vi "Instrument_Setup.vi"() -> ()   [LabVIEW 2016]
uses:
  sub_vi-s/Equipment/Oxford Software/Oxsoft/PSSUBS.LLB/PSIO.ctl
  sub_vi-s/Equipment/Oxford Software/Oxsoft/BUSGEN.LLB/OxfordAddress.ctl
  sub_vi-s/Equipment/Oxford Software/Oxsoft/ITCSUBS.LLB/ITCIO.ctl
  sub_vi-s/Equipment/Oxford Software/Oxsoft/ITCSUBS.LLB/ITCVersion.ctl
  sub_vi-s/Equipment/Oxford Software/Oxsoft/PSAPPS.LLB/PSSetupArray.ctl
  sub_vi-s/Equipment/Oxford Software/Oxsoft/PSAPPS.LLB/PSSetup.ctl
  sub_vi-s/Equipment/Oxford Software/Oxsoft/ITCAPPS.LLB/ITCSetup.ctl
  sub_vi-s/Equipment/Oxford Software/Oxsoft/LCSUBS.LLB/LambdaSetup.ctl
  sub_vi-s/Equipment/Oxford Software/Oxsoft/Ilmapps.llb/ILMSetup.ctl
panel:
  in  "Registerkarte":T1(tab)=enum."Keithley 6221"
  in  "Insert":string(combo)="VTI"
  in  "Instrument":string(combo)="Sweet 16"
  in  "Temperature control":bool
  in  "Set-Lockin-Sens":u16(ring) items=["Command File", "Auto", "Status Monitor"]
  in  "Logfile folder":path=path "D:/Cryostat Software/Logfiles"
  in  "16 T":bool
  in  "AH 2500":bool
  in  "Set magnet persistent":bool
  in  "Keithley 6221":bool
  in  "readout (s)":dbl=1.0 min=0.0 format="%#_6f"
  in  "LS372 mitloggen":bool
  in  "Stepmodus":enum16{"linear", "1/x", "Logx"}(ring)
  in  "LS370 mitloggen":bool
  in  "Initializiation-File-Folder":path=path "D:/Messdaten/Init-Files"
  in  "Command-File":path=path "D:/Cryostat Software/CryoTUM-V1.0/Command-File.txt"
  in  "Datafile-Folder":path=path "D:/Messdaten"
  in  "Keithley":bool
  in  "Lock In #3":bool
  in  "Lock In #2":bool
  in  "Lock In #1":bool
  in  "Heater &\nNeedle Valve":bool
  in  "Hall contact dist. (mm)":string="1"
  in  "Sample thickness (mm)":string="1"
  in  "Contact dist. (mm)":string="1"
  in  "Sample width (mm)":string="1"
  in  "Wait for LS340":bool
  in  "Dropping Resistance [kOhm]":string="1"
  in  "Amplification":string="1"
  in  "Measure for time of CC skript\nat each field step point":bool
  in  "Sample":string
  in  "User":string
  in  "seconds to wait at each\ncurrent step in a I-step sweep":dbl=20.0
  in  "seconds to wait after needle\nvalve was set from auto to\nmanual":dbl=60.0
  in  "LS340 mitloggen":bool
  in  "seconds to wait at each\nfield step in a step sweep":dbl=20.0
  in  "minutes for CC\nto run":dbl=60.0
  in  "seconds-to-wait-after-\nLock-In-initialization":dbl=20.0
  in  "Autoshutdown":bool
  in  "Sweep-Tolerance-\nTemperature":dbl=0.1
  in  "Sweep-Tolerance-\nMagnetic-Field":dbl=1e-06
  in  "AH 2700":bool
  in  "Torque \nMeasurem.":bool
  in  "Keithley 4R":bool
  in  "Update Lockins":bool
  in  "Auto-Sens-Threshold (%)":dbl=1.0
  in  "Lock In 3 GPIB address":string="10"
  in  "Lock-in Readout time":dbl=1.0
  in  "Lock In 2 time constant":T2={"time constant\n(10 µs : 0) "=12, "slope (6 dB/oct)"=3} {"slope (6 dB/oct)" items=["6 dB/oct", "12 dB/oct", "18 dB/oct", "24 dB/oct"]; "time constant\n(10 µs : 0)" items=["10 µs", "30 µs", "100 µs", "300 µs", "1 ms", "3 ms", "10 ms", "30 ms", "100 ms", "300 ms", "1 s", "3 s", "10 s", "30 s", "100 s", "300 s", "1 ks", "3 ks", "10 ks", "30 ks"]}
  in  "Lock In 2 sync":T3 {"line filter\n(off:0)" items=["OFF", "line", "2 x line", "both"]}
  in  "Lock In 2 sensitivity":T4={"sensitivity\n2nV/fA"=0, "dyn reserve\n(low noise:2)"=2, "ref. phase"=0.0, "automeasure"=FALSE} {"sensitivity\n2nV/fA" items=["2 nV/fA", "5 nV/fA", "10 nV/fA", "20 nV/fA", "50 nV/fA", "100 nV/fA", "200 nV/fA", "500 nV/fA", "1 µV /pA", "2 µV/pA", "5 µV/pA", "10 µV/pA", "20 µV/pA", "50 µV/pA", "100 µV/pA", "200 µV/pA", "500 µV/pA", "1 mV/nA", "2 mV/nA", "5 mV/nA", "10 mV/nA", "20 mV/nA", "50 mV/nA", "100 mV/nA", "200 mV/nA", "500 mV/nA", "1 V/µA"]; "dyn reserve\n(low noise:2)" scale=0.0..2.0 scale format="%.2f"; "ref. phase" format="%.2f"}
  in  "Lock In 2 reference":T5={"ref. source"=FALSE, "osc.harm# "=1, "osc. freq"=0.001, "osc. ampl."=0.004, "ref. trigger"=0} {"ref. trigger" items=["sine", "pos edge", "neg edge"]; "osc.harm#" min=1 max=19999; "osc. ampl." format="%.3f"; "osc. freq" format="%.3f"}
  in  "Lock In 2 off. & exp.":T6 {"expand" items=["none", "x 10", "x 100"]; "offset" format="%.2f"; "off. & exp." items=["X", "Y", "R"]}
  in  "Lock In 2 input":T7={"input"=1, "ground"=FALSE, "couple"=TRUE} {"input" items=["A", "A-B", "I (1 M gain)", "I (100 M gain)"]}
  in  "Lock In 2 GPIB address":string="9"
  in  "Lock In 2 channel 2":T8={" display"=0, " ratio"=0, "output"=1} {"output" items=["display", "Y"]; "ratio" items=["none", "aux in 3", "aux in 4"]; "display" items=["Y", "@", "Y Noise", "Aux In 3", "Aux In 4"]}
  in  "Lock In 2 channel 1":T8={" display"=0, " ratio"=0, "output"=1} {"output" items=["display", "X"]; "ratio" items=["none", "aux in 1", "aux in 2"]; "display" items=["X", "R", "X Noise", "Aux In 1", "Aux In 2"]}
  in  "Lock In 1 time constant":T2={"time constant\n(10 µs : 0) "=12, "slope (6 dB/oct)"=3} {"slope (6 dB/oct)" items=["6 dB/oct", "12 dB/oct", "18 dB/oct", "24 dB/oct"]; "time constant\n(10 µs : 0)" items=["10 µs", "30 µs", "100 µs", "300 µs", "1 ms", "3 ms", "10 ms", "30 ms", "100 ms", "300 ms", "1 s", "3 s", "10 s", "30 s", "100 s", "300 s", "1 ks", "3 ks", "10 ks", "30 ks"]}
  in  "Lock In 1 sync":T3 {"line filter\n(off:0)" items=["OFF", "line", "2 x line", "both"]}
  in  "Lock In 1 sensitivity":T4={"sensitivity\n2nV/fA"=0, "dyn reserve\n(low noise:2)"=2, "ref. phase"=0.0, "automeasure"=FALSE} {"sensitivity\n2nV/fA" items=["2 nV/fA", "5 nV/fA", "10 nV/fA", "20 nV/fA", "50 nV/fA", "100 nV/fA", "200 nV/fA", "500 nV/fA", "1 µV /pA", "2 µV/pA", "5 µV/pA", "10 µV/pA", "20 µV/pA", "50 µV/pA", "100 µV/pA", "200 µV/pA", "500 µV/pA", "1 mV/nA", "2 mV/nA", "5 mV/nA", "10 mV/nA", "20 mV/nA", "50 mV/nA", "100 mV/nA", "200 mV/nA", "500 mV/nA", "1 V/µA"]; "dyn reserve\n(low noise:2)" scale=0.0..2.0 scale format="%.2f"; "ref. phase" format="%.2f"}
  in  "Lock In 1 reference":T5={"ref. source"=TRUE, "osc.harm# "=1, "osc. freq"=22.08, "osc. ampl."=5.0, "ref. trigger"=0} {"ref. trigger" items=["sine", "pos edge", "neg edge"]; "osc.harm#" min=1 max=19999; "osc. ampl." format="%.3f"; "osc. freq" format="%.3f"}
  in  "Lock In 1 off. & exp.":T6 {"expand" items=["none", "x 10", "x 100"]; "offset" format="%.2f"; "off. & exp." items=["X", "Y", "R"]}
  in  "Lock In 1 input":T7={"input"=1, "ground"=FALSE, "couple"=TRUE} {"input" items=["A", "A-B", "I (1 M gain)", "I (100 M gain)"]}
  in  "Lock In 1 GPIB address":string="8"
  in  "Lock In 1 channel 2":T8={" display"=0, " ratio"=0, "output"=1} {"output" items=["display", "Y"]; "ratio" items=["none", "aux in 3", "aux in 4"]; "display" items=["Y", "@", "Y Noise", "Aux In 3", "Aux In 4"]}
  in  "Lock In 1 channel 1":T8={" display"=0, " ratio"=0, "output"=1} {"output" items=["display", "X"]; "ratio" items=["none", "aux in 1", "aux in 2"]; "display" items=["X", "R", "X Noise", "Aux In 1", "Aux In 2"]}
  in  "Keithley connected?":bool
  in  "VISA Keithley":refnum<visa-resource-name>="GPIB0::24::INSTR"
  in  "Source Mode  (1: Current)":u16(ring)=1 items=["Current"=1, "Voltage"=0]
  in  "Compliance  Level (3.0 V)":dbl=42.0
  in  "Enable Resistance Auto Range (T:Enable)":bool=TRUE
  in  "Enable Current Auto Range (T:Enable) 2":bool=TRUE
  in  "Enable Voltage Auto Range (T:Enable)":bool=TRUE
  in  "Resistance Manual Range (1.0)":dbl=1.0
  in  "Current Manual Range (1.0)":dbl=1.0
  in  "Voltage Manual Range (1.0)":dbl=1.0
  in  "6221 Current is given as RMS?":bool
  in  "Set-Keithley-6221":u16(ring) items=["Command File", "Status Monitor"]
  in  "Frequency (Hz)":dbl=0.001
  in  "Phase Marker (deg)":dbl
  in  "Trig Link Line":i32=3 min=0 step=1
  in  "Offset (A)":dbl
  in  "Phase Marker?":bool=TRUE
  in  "Amplitude (A)":dbl=0.001 format="%.6f"
  in  "VISA resource name 6221":refnum<visa-resource-name>="GPIB0::22::INSTR"
  in  "Keithley 6221 connected?":bool
  in  "maximaler Strom [mA]":i32=700 min=0 max=1500 step=1
  in  "maximale Positionierungsgeschwindigkeit":i32=115 min=0 max=2047 step=1
  in  "Mikro-Schrittweite":i32=6 min=0 max=6 step=1
  in  "Maximale Beschleunigung":i32=500 min=0 max=2047 step=1
  in  "VISA Torque Motor":refnum<visa-resource-name>="COM5"
  in  "baud rate":u32=9600
  in  "data bits":u16=8 min=5 max=8 step=1
  in  "parity":u16(ring) items=["None", "Odd", "Even", "Mark", "Space"]
  in  "stop bits":u16(ring)=10 items=["1.0"=10, "1.5"=15, "2.0"=20]
  in  "flow control":u16(ring) items=["None"=0, "XON/XOFF"=1, "RTS/CTS"=2, "DTR/DSR"=4]
  in  "Num Monitor":dbl=5000.0 min=0.0 format="%#_6f"
  in  "Sorb Heater Resistance (Analog Out 1)":dbl=285.0 min=0.0 format="%#_6f"
  in  "MC Heater Resistance":dbl=500.0 min=0.0 format="%#_6f"
  in  "Still Heater Resistance (Analog  Out  2)":dbl=500.0 min=0.0 format="%#_6f"
  in  "Excitation Range CH3 (11: 632 mV / 316 nA)":u16(ring)=5 items=["2.00 uV / 1.00 pA", "6.32 uV / 3.16 pA", "20.0 uV / 10.0 pA", "63.2 uV / 31.6 pA", "200 uV / 100 pA", "632 uV / 316 pA", "2.00 mV / 1.00 nA", "6.32 mV / 3.16 nA", "20.0 mV / 10.0 nA", "63.2 mV / 31.6 nA", "200 mV / 100 nA", "632 mV / 316 nA", "1.00 uA", "3.16 uA", "10.0 uA", "31.6 uA", "100 uA", "316 uA", "1.00 mA", "3.16 mA", "10.0 mA", "31.6 mA"]
  in  "Scan Dwell Time  TC (10)":dbl=10.0 min=1.0 max=200.0 step=1.0
  in  "Lakeshore 370 #1":bool
  in  "Calibration 1":i32=4 min=0 max=16 step=1
  in  "Autorange Ch 1":bool
  in  "Channel 1":i32=4 min=0 max=16 step=1
  in  "Resistance Range CH1(21: 63.2 MOhm)":u16(ring)=13 items=["2.00 mOhm", "6.32 mOhm", "20.0 mOhm", "63.2 mOhm", "200 mOhm", "632 mOhm", "2.00 Ohm", "6.32 Ohm", "20.0 Ohm", "63.2 Ohm", "200 Ohm", "632 Ohm", "2.00 kOhm", "6.32 kOhm", "20.0 kOhm", "63.2 kOhm", "200 kOhm", "632 kOhm", "2.00 MOhm", "6.32 MOhm", "20.0 MOhm", "63.2 MOhm"]
  in  "Excitation Range CH1 (11: 632 mV / 316 nA)":u16(ring)=5 items=["2.00 uV / 1.00 pA", "6.32 uV / 3.16 pA", "20.0 uV / 10.0 pA", "63.2 uV / 31.6 pA", "200 uV / 100 pA", "632 uV / 316 pA", "2.00 mV / 1.00 nA", "6.32 mV / 3.16 nA", "20.0 mV / 10.0 nA", "63.2 mV / 31.6 nA", "200 mV / 100 nA", "632 mV / 316 nA", "1.00 uA", "3.16 uA", "10.0 uA", "31.6 uA", "100 uA", "316 uA", "1.00 mA", "3.16 mA", "10.0 mA", "31.6 mA"]
  in  "Lakeshore 370 # TC":bool=TRUE
  in  "Lakeshore 370 #9":bool
  in  "Lakeshore 370 #8":bool
  in  "Lakeshore 370 #7":bool
  in  "Lakeshore 370 #6":bool
  in  "Calibration 5":i32=1 min=0 max=16 step=1
  in  "Channel 5":i32=11 min=0 max=16 step=1
  in  "Autorange Ch 5":bool
  in  "Resistance Range CH5 (21: 63.2 MOhm)":u16(ring)=21 items=["2.00 mOhm", "6.32 mOhm", "20.0 mOhm", "63.2 mOhm", "200 mOhm", "632 mOhm", "2.00 Ohm", "6.32 Ohm", "20.0 Ohm", "63.2 Ohm", "200 Ohm", "632 Ohm", "2.00 kOhm", "6.32 kOhm", "20.0 kOhm", "63.2 kOhm", "200 kOhm", "632 kOhm", "2.00 MOhm", "6.32 MOhm", "20.0 MOhm", "63.2 MOhm"]
  in  "Excitation Range CH 5 (11: 632 mV / 316 nA)":u16(ring)=11 items=["2.00 uV / 1.00 pA", "6.32 uV / 3.16 pA", "20.0 uV / 10.0 pA", "63.2 uV / 31.6 pA", "200 uV / 100 pA", "632 uV / 316 pA", "2.00 mV / 1.00 nA", "6.32 mV / 3.16 nA", "20.0 mV / 10.0 nA", "63.2 mV / 31.6 nA", "200 mV / 100 nA", "632 mV / 316 nA", "1.00 uA", "3.16 uA", "10.0 uA", "31.6 uA", "100 uA", "316 uA", "1.00 mA", "3.16 mA", "10.0 mA", "31.6 mA"]
  in  "Calibration 7":i32=1 min=0 max=16 step=1
  in  "Channel 7":i32=7 min=0 max=16 step=1
  in  "Autorange Ch 7":bool
  in  "Resistance Range CH7 (21: 63.2 MOhm)":u16(ring)=21 items=["2.00 mOhm", "6.32 mOhm", "20.0 mOhm", "63.2 mOhm", "200 mOhm", "632 mOhm", "2.00 Ohm", "6.32 Ohm", "20.0 Ohm", "63.2 Ohm", "200 Ohm", "632 Ohm", "2.00 kOhm", "6.32 kOhm", "20.0 kOhm", "63.2 kOhm", "200 kOhm", "632 kOhm", "2.00 MOhm", "6.32 MOhm", "20.0 MOhm", "63.2 MOhm"]
  in  "Excitation Range CH7 (11: 632 mV / 316 nA)":u16(ring)=11 items=["2.00 uV / 1.00 pA", "6.32 uV / 3.16 pA", "20.0 uV / 10.0 pA", "63.2 uV / 31.6 pA", "200 uV / 100 pA", "632 uV / 316 pA", "2.00 mV / 1.00 nA", "6.32 mV / 3.16 nA", "20.0 mV / 10.0 nA", "63.2 mV / 31.6 nA", "200 mV / 100 nA", "632 mV / 316 nA", "1.00 uA", "3.16 uA", "10.0 uA", "31.6 uA", "100 uA", "316 uA", "1.00 mA", "3.16 mA", "10.0 mA", "31.6 mA"]
  in  "Calibration 4":i32=1 min=0 max=16 step=1
  in  "Channel 4":i32=1 min=0 max=16 step=1
  in  "Autorange Ch 4":bool
  in  "Resistance Range CH4 (21: 63.2 MOhm)":u16(ring)=12 items=["2.00 mOhm", "6.32 mOhm", "20.0 mOhm", "63.2 mOhm", "200 mOhm", "632 mOhm", "2.00 Ohm", "6.32 Ohm", "20.0 Ohm", "63.2 Ohm", "200 Ohm", "632 Ohm", "2.00 kOhm", "6.32 kOhm", "20.0 kOhm", "63.2 kOhm", "200 kOhm", "632 kOhm", "2.00 MOhm", "6.32 MOhm", "20.0 MOhm", "63.2 MOhm"]
  in  "Excitation Range CH4 (11: 632 mV / 316 nA)":u16(ring)=5 items=["2.00 uV / 1.00 pA", "6.32 uV / 3.16 pA", "20.0 uV / 10.0 pA", "63.2 uV / 31.6 pA", "200 uV / 100 pA", "632 uV / 316 pA", "2.00 mV / 1.00 nA", "6.32 mV / 3.16 nA", "20.0 mV / 10.0 nA", "63.2 mV / 31.6 nA", "200 mV / 100 nA", "632 mV / 316 nA", "1.00 uA", "3.16 uA", "10.0 uA", "31.6 uA", "100 uA", "316 uA", "1.00 mA", "3.16 mA", "10.0 mA", "31.6 mA"]
  in  "Calibration 6":i32=1 min=0 max=16 step=1
  in  "Channel 6":i32=6 min=0 max=16 step=1
  in  "Autorange Ch 6":bool
  in  "Resistance Range CH6(21: 63.2 MOhm)":u16(ring)=12 items=["2.00 mOhm", "6.32 mOhm", "20.0 mOhm", "63.2 mOhm", "200 mOhm", "632 mOhm", "2.00 Ohm", "6.32 Ohm", "20.0 Ohm", "63.2 Ohm", "200 Ohm", "632 Ohm", "2.00 kOhm", "6.32 kOhm", "20.0 kOhm", "63.2 kOhm", "200 kOhm", "632 kOhm", "2.00 MOhm", "6.32 MOhm", "20.0 MOhm", "63.2 MOhm"]
  in  "Excitation Range CH6 (11: 632 mV / 316 nA)":u16(ring)=5 items=["2.00 uV / 1.00 pA", "6.32 uV / 3.16 pA", "20.0 uV / 10.0 pA", "63.2 uV / 31.6 pA", "200 uV / 100 pA", "632 uV / 316 pA", "2.00 mV / 1.00 nA", "6.32 mV / 3.16 nA", "20.0 mV / 10.0 nA", "63.2 mV / 31.6 nA", "200 mV / 100 nA", "632 mV / 316 nA", "1.00 uA", "3.16 uA", "10.0 uA", "31.6 uA", "100 uA", "316 uA", "1.00 mA", "3.16 mA", "10.0 mA", "31.6 mA"]
  in  "Temperature control channel":i32=5 min=0 max=16 step=1
  in  "Calibration 9":i32=1 min=0 max=16 step=1
  in  "Channel 9":i32=9 min=0 max=16 step=1
  in  "Autorange Ch 9":bool
  in  "Resistance Range CH9(21: 63.2 MOhm)":u16(ring)=21 items=["2.00 mOhm", "6.32 mOhm", "20.0 mOhm", "63.2 mOhm", "200 mOhm", "632 mOhm", "2.00 Ohm", "6.32 Ohm", "20.0 Ohm", "63.2 Ohm", "200 Ohm", "632 Ohm", "2.00 kOhm", "6.32 kOhm", "20.0 kOhm", "63.2 kOhm", "200 kOhm", "632 kOhm", "2.00 MOhm", "6.32 MOhm", "20.0 MOhm", "63.2 MOhm"]
  in  "Excitation Range CH9(11: 632 mV / 316 nA)":u16(ring)=11 items=["2.00 uV / 1.00 pA", "6.32 uV / 3.16 pA", "20.0 uV / 10.0 pA", "63.2 uV / 31.6 pA", "200 uV / 100 pA", "632 uV / 316 pA", "2.00 mV / 1.00 nA", "6.32 mV / 3.16 nA", "20.0 mV / 10.0 nA", "63.2 mV / 31.6 nA", "200 mV / 100 nA", "632 mV / 316 nA", "1.00 uA", "3.16 uA", "10.0 uA", "31.6 uA", "100 uA", "316 uA", "1.00 mA", "3.16 mA", "10.0 mA", "31.6 mA"]
  in  "Calibration 8":i32=1 min=0 max=16 step=1
  in  "Channel 8":i32=8 min=0 max=16 step=1
  in  "Autorange Ch 8":bool
  in  "Resistance Range CH8(21: 63.2 MOhm)":u16(ring)=21 items=["2.00 mOhm", "6.32 mOhm", "20.0 mOhm", "63.2 mOhm", "200 mOhm", "632 mOhm", "2.00 Ohm", "6.32 Ohm", "20.0 Ohm", "63.2 Ohm", "200 Ohm", "632 Ohm", "2.00 kOhm", "6.32 kOhm", "20.0 kOhm", "63.2 kOhm", "200 kOhm", "632 kOhm", "2.00 MOhm", "6.32 MOhm", "20.0 MOhm", "63.2 MOhm"]
  in  "Excitation Range CH8 (11: 632 mV / 316 nA)":u16(ring)=11 items=["2.00 uV / 1.00 pA", "6.32 uV / 3.16 pA", "20.0 uV / 10.0 pA", "63.2 uV / 31.6 pA", "200 uV / 100 pA", "632 uV / 316 pA", "2.00 mV / 1.00 nA", "6.32 mV / 3.16 nA", "20.0 mV / 10.0 nA", "63.2 mV / 31.6 nA", "200 mV / 100 nA", "632 mV / 316 nA", "1.00 uA", "3.16 uA", "10.0 uA", "31.6 uA", "100 uA", "316 uA", "1.00 mA", "3.16 mA", "10.0 mA", "31.6 mA"]
  in  "Autoscan":bool
  in  "Calibration TC":i32=5 min=0 max=16 step=1
  in  "Calibration 3":i32=3 min=0 max=16 step=1
  in  "Calibration 2":i32=2 min=0 max=16 step=1
  in  "Channel 3":i32=3 min=0 max=16 step=1
  in  "Channel 2":i32=2 min=0 max=16 step=1
  in  "Autorange Ch 3":bool
  in  "Autorange Ch 2":bool
  in  "Autorange Ch TC":bool
  in  "Excitation Range CH2 (11: 632 mV / 316 nA)":u16(ring)=5 items=["2.00 uV / 1.00 pA", "6.32 uV / 3.16 pA", "20.0 uV / 10.0 pA", "63.2 uV / 31.6 pA", "200 uV / 100 pA", "632 uV / 316 pA", "2.00 mV / 1.00 nA", "6.32 mV / 3.16 nA", "20.0 mV / 10.0 nA", "63.2 mV / 31.6 nA", "200 mV / 100 nA", "632 mV / 316 nA", "1.00 uA", "3.16 uA", "10.0 uA", "31.6 uA", "100 uA", "316 uA", "1.00 mA", "3.16 mA", "10.0 mA", "31.6 mA"]
  in  "Resistance Range CH3 (21: 63.2 MOhm)":u16(ring)=12 items=["2.00 mOhm", "6.32 mOhm", "20.0 mOhm", "63.2 mOhm", "200 mOhm", "632 mOhm", "2.00 Ohm", "6.32 Ohm", "20.0 Ohm", "63.2 Ohm", "200 Ohm", "632 Ohm", "2.00 kOhm", "6.32 kOhm", "20.0 kOhm", "63.2 kOhm", "200 kOhm", "632 kOhm", "2.00 MOhm", "6.32 MOhm", "20.0 MOhm", "63.2 MOhm"]
  in  "Resistance Range CH2 (21: 63.2 MOhm)":u16(ring)=12 items=["2.00 mOhm", "6.32 mOhm", "20.0 mOhm", "63.2 mOhm", "200 mOhm", "632 mOhm", "2.00 Ohm", "6.32 Ohm", "20.0 Ohm", "63.2 Ohm", "200 Ohm", "632 Ohm", "2.00 kOhm", "6.32 kOhm", "20.0 kOhm", "63.2 kOhm", "200 kOhm", "632 kOhm", "2.00 MOhm", "6.32 MOhm", "20.0 MOhm", "63.2 MOhm"]
  in  "Resistance Range TC (21: 63.2 MOhm)":u16(ring)=15 items=["2.00 mOhm", "6.32 mOhm", "20.0 mOhm", "63.2 mOhm", "200 mOhm", "632 mOhm", "2.00 Ohm", "6.32 Ohm", "20.0 Ohm", "63.2 Ohm", "200 Ohm", "632 Ohm", "2.00 kOhm", "6.32 kOhm", "20.0 kOhm", "63.2 kOhm", "200 kOhm", "632 kOhm", "2.00 MOhm", "6.32 MOhm", "20.0 MOhm", "63.2 MOhm"]
  in  "Excitation Range TC (11: 632 mV / 316 nA)":u16(ring)=5 items=["2.00 uV / 1.00 pA", "6.32 uV / 3.16 pA", "20.0 uV / 10.0 pA", "63.2 uV / 31.6 pA", "200 uV / 100 pA", "632 uV / 316 pA", "2.00 mV / 1.00 nA", "6.32 mV / 3.16 nA", "20.0 mV / 10.0 nA", "63.2 mV / 31.6 nA", "200 mV / 100 nA", "632 mV / 316 nA", "1.00 uA", "3.16 uA", "10.0 uA", "31.6 uA", "100 uA", "316 uA", "1.00 mA", "3.16 mA", "10.0 mA", "31.6 mA"]
  in  "Change Pause Time (3)":dbl=3.0 min=3.0 max=200.0 step=1.0
  in  "Excitation On/Off (T: Excitation ON)":bool=TRUE
  in  "Configure (F:Don't Config)":bool
  in  "Channel On/Off (T: Channel ON)":bool=TRUE
  in  "Temperature Coefficient (0: Negative)":u16(ring) items=["Negative", "Positive"]
  in  "Excitation Mode (0: Voltage)":u16(ring) items=["Voltage", "Current"]
  in  "Scan Dwell Time (10)":dbl=10.0 min=1.0 max=200.0 step=1.0
  in  "VISA session LS1":refnum<visa-resource-name>="GPIB0::17::INSTR"
  in  "Lakeshore 370 #2":bool
  in  "Lakeshore 370 #3":bool
  in  "Lakeshore 370 #4":bool
  in  "Lakeshore 370 #5":bool
  in  "LS372 Filter Time":dbl=10.0 min=1.0 max=200.0 step=1.0
  in  "LS372 Filter Window":dbl=40.0 min=1.0 max=200.0 step=1.0
  in  "LS372 Filter":bool=TRUE
  in  "Excitation Range2-6":u16(ring)=5 items=["2.00 uV / 1.00 pA"=1, "6.32 uV / 3.16 pA"=2, "20.0 uV / 10.0 pA"=3, "63.2 uV / 31.6 pA"=4, "200 uV / 100 pA"=5, "632 uV / 316 pA"=6, "2.00 mV / 1.00 nA"=7, "6.32 mV / 3.16 nA"=8, "20.0 mV / 10.0 nA"=9, "63.2 mV / 31.6 nA"=10, "200 mV / 100 nA"=11, "632 mV / 316 nA"=12, "1.00 uA"=13, "3.16 uA"=14, "10.0 uA"=15, "31.6 uA"=16, "100 uA"=17, "316 uA"=18, "1.00 mA"=19, "3.16 mA"=20, "10.0 mA"=21, "31.6 mA"=22]
  in  "Excitation Range2-5":u16(ring)=5 items=["2.00 uV / 1.00 pA"=1, "6.32 uV / 3.16 pA"=2, "20.0 uV / 10.0 pA"=3, "63.2 uV / 31.6 pA"=4, "200 uV / 100 pA"=5, "632 uV / 316 pA"=6, "2.00 mV / 1.00 nA"=7, "6.32 mV / 3.16 nA"=8, "20.0 mV / 10.0 nA"=9, "63.2 mV / 31.6 nA"=10, "200 mV / 100 nA"=11, "632 mV / 316 nA"=12, "1.00 uA"=13, "3.16 uA"=14, "10.0 uA"=15, "31.6 uA"=16, "100 uA"=17, "316 uA"=18, "1.00 mA"=19, "3.16 mA"=20, "10.0 mA"=21, "31.6 mA"=22]
  in  "Excitation Range2-4":u16(ring)=5 items=["2.00 uV / 1.00 pA"=1, "6.32 uV / 3.16 pA"=2, "20.0 uV / 10.0 pA"=3, "63.2 uV / 31.6 pA"=4, "200 uV / 100 pA"=5, "632 uV / 316 pA"=6, "2.00 mV / 1.00 nA"=7, "6.32 mV / 3.16 nA"=8, "20.0 mV / 10.0 nA"=9, "63.2 mV / 31.6 nA"=10, "200 mV / 100 nA"=11, "632 mV / 316 nA"=12, "1.00 uA"=13, "3.16 uA"=14, "10.0 uA"=15, "31.6 uA"=16, "100 uA"=17, "316 uA"=18, "1.00 mA"=19, "3.16 mA"=20, "10.0 mA"=21, "31.6 mA"=22]
  in  "Excitation Range2-3":u16(ring)=5 items=["2.00 uV / 1.00 pA"=1, "6.32 uV / 3.16 pA"=2, "20.0 uV / 10.0 pA"=3, "63.2 uV / 31.6 pA"=4, "200 uV / 100 pA"=5, "632 uV / 316 pA"=6, "2.00 mV / 1.00 nA"=7, "6.32 mV / 3.16 nA"=8, "20.0 mV / 10.0 nA"=9, "63.2 mV / 31.6 nA"=10, "200 mV / 100 nA"=11, "632 mV / 316 nA"=12, "1.00 uA"=13, "3.16 uA"=14, "10.0 uA"=15, "31.6 uA"=16, "100 uA"=17, "316 uA"=18, "1.00 mA"=19, "3.16 mA"=20, "10.0 mA"=21, "31.6 mA"=22]
  in  "Excitation Range2-2":u16(ring)=5 items=["2.00 uV / 1.00 pA"=1, "6.32 uV / 3.16 pA"=2, "20.0 uV / 10.0 pA"=3, "63.2 uV / 31.6 pA"=4, "200 uV / 100 pA"=5, "632 uV / 316 pA"=6, "2.00 mV / 1.00 nA"=7, "6.32 mV / 3.16 nA"=8, "20.0 mV / 10.0 nA"=9, "63.2 mV / 31.6 nA"=10, "200 mV / 100 nA"=11, "632 mV / 316 nA"=12, "1.00 uA"=13, "3.16 uA"=14, "10.0 uA"=15, "31.6 uA"=16, "100 uA"=17, "316 uA"=18, "1.00 mA"=19, "3.16 mA"=20, "10.0 mA"=21, "31.6 mA"=22]
  in  "Excitation Range2-1":u16(ring)=5 items=["2.00 uV / 1.00 pA"=1, "6.32 uV / 3.16 pA"=2, "20.0 uV / 10.0 pA"=3, "63.2 uV / 31.6 pA"=4, "200 uV / 100 pA"=5, "632 uV / 316 pA"=6, "2.00 mV / 1.00 nA"=7, "6.32 mV / 3.16 nA"=8, "20.0 mV / 10.0 nA"=9, "63.2 mV / 31.6 nA"=10, "200 mV / 100 nA"=11, "632 mV / 316 nA"=12, "1.00 uA"=13, "3.16 uA"=14, "10.0 uA"=15, "31.6 uA"=16, "100 uA"=17, "316 uA"=18, "1.00 mA"=19, "3.16 mA"=20, "10.0 mA"=21, "31.6 mA"=22]
  in  "Resistance Range2-6":u16(ring)=17 items=["2.00 mOhm"=1, "6.32 mOhm"=2, "20.0 mOhm"=3, "63.2 mOhm"=4, "200 mOhm"=5, "632 mOhm"=6, "2.00 Ohm"=7, "6.32 Ohm"=8, "20.0 Ohm"=9, "63.2 Ohm"=10, "200 Ohm"=11, "632 Ohm"=12, "2.00 kOhm"=13, "6.32 kOhm"=14, "20.0 kOhm"=15, "63.2 kOhm"=16, "200 kOhm"=17, "632 kOhm"=18, "2.00 MOhm"=19, "6.32 MOhm"=20, "20.0 MOhm"=21, "63.2 MOhm"=22]
  in  "Resistance Range2-5":u16(ring)=17 items=["2.00 mOhm"=1, "6.32 mOhm"=2, "20.0 mOhm"=3, "63.2 mOhm"=4, "200 mOhm"=5, "632 mOhm"=6, "2.00 Ohm"=7, "6.32 Ohm"=8, "20.0 Ohm"=9, "63.2 Ohm"=10, "200 Ohm"=11, "632 Ohm"=12, "2.00 kOhm"=13, "6.32 kOhm"=14, "20.0 kOhm"=15, "63.2 kOhm"=16, "200 kOhm"=17, "632 kOhm"=18, "2.00 MOhm"=19, "6.32 MOhm"=20, "20.0 MOhm"=21, "63.2 MOhm"=22]
  in  "Resistance Range2-4":u16(ring)=17 items=["2.00 mOhm"=1, "6.32 mOhm"=2, "20.0 mOhm"=3, "63.2 mOhm"=4, "200 mOhm"=5, "632 mOhm"=6, "2.00 Ohm"=7, "6.32 Ohm"=8, "20.0 Ohm"=9, "63.2 Ohm"=10, "200 Ohm"=11, "632 Ohm"=12, "2.00 kOhm"=13, "6.32 kOhm"=14, "20.0 kOhm"=15, "63.2 kOhm"=16, "200 kOhm"=17, "632 kOhm"=18, "2.00 MOhm"=19, "6.32 MOhm"=20, "20.0 MOhm"=21, "63.2 MOhm"=22]
  in  "Resistance Range2-2":u16(ring)=15 items=["2.00 mOhm"=1, "6.32 mOhm"=2, "20.0 mOhm"=3, "63.2 mOhm"=4, "200 mOhm"=5, "632 mOhm"=6, "2.00 Ohm"=7, "6.32 Ohm"=8, "20.0 Ohm"=9, "63.2 Ohm"=10, "200 Ohm"=11, "632 Ohm"=12, "2.00 kOhm"=13, "6.32 kOhm"=14, "20.0 kOhm"=15, "63.2 kOhm"=16, "200 kOhm"=17, "632 kOhm"=18, "2.00 MOhm"=19, "6.32 MOhm"=20, "20.0 MOhm"=21, "63.2 MOhm"=22]
  in  "Resistance Range2-3":u16(ring)=17 items=["2.00 mOhm"=1, "6.32 mOhm"=2, "20.0 mOhm"=3, "63.2 mOhm"=4, "200 mOhm"=5, "632 mOhm"=6, "2.00 Ohm"=7, "6.32 Ohm"=8, "20.0 Ohm"=9, "63.2 Ohm"=10, "200 Ohm"=11, "632 Ohm"=12, "2.00 kOhm"=13, "6.32 kOhm"=14, "20.0 kOhm"=15, "63.2 kOhm"=16, "200 kOhm"=17, "632 kOhm"=18, "2.00 MOhm"=19, "6.32 MOhm"=20, "20.0 MOhm"=21, "63.2 MOhm"=22]
  in  "Resistance Range2-1":u16(ring)=15 items=["2.00 mOhm"=1, "6.32 mOhm"=2, "20.0 mOhm"=3, "63.2 mOhm"=4, "200 mOhm"=5, "632 mOhm"=6, "2.00 Ohm"=7, "6.32 Ohm"=8, "20.0 Ohm"=9, "63.2 Ohm"=10, "200 Ohm"=11, "632 Ohm"=12, "2.00 kOhm"=13, "6.32 kOhm"=14, "20.0 kOhm"=15, "63.2 kOhm"=16, "200 kOhm"=17, "632 kOhm"=18, "2.00 MOhm"=19, "6.32 MOhm"=20, "20.0 MOhm"=21, "63.2 MOhm"=22]
  in  "Channel2-4":u16(ring)=3 items=["1"=1, "2"=2, "3"=3, "4"=4, "5"=5, "6"=6, "7"=7, "8"=8, "9"=9, "10"=10, "11"=11, "12"=12, "13"=13, "14"=14, "15"=15, "16"=16, "A (Control Input)"=17]
  in  "Channel2-6":u16(ring)=5 items=["1"=1, "2"=2, "3"=3, "4"=4, "5"=5, "6"=6, "7"=7, "8"=8, "9"=9, "10"=10, "11"=11, "12"=12, "13"=13, "14"=14, "15"=15, "16"=16, "A (Control Input)"=17]
  in  "Channel2-5":u16(ring)=4 items=["1"=1, "2"=2, "3"=3, "4"=4, "5"=5, "6"=6, "7"=7, "8"=8, "9"=9, "10"=10, "11"=11, "12"=12, "13"=13, "14"=14, "15"=15, "16"=16, "A (Control Input)"=17]
  in  "Channel2-3":u16(ring)=2 items=["1"=1, "2"=2, "3"=3, "4"=4, "5"=5, "6"=6, "7"=7, "8"=8, "9"=9, "10"=10, "11"=11, "12"=12, "13"=13, "14"=14, "15"=15, "16"=16, "A (Control Input)"=17]
  in  "Channel2-1":u16(ring)=17 items=["1"=1, "2"=2, "3"=3, "4"=4, "5"=5, "6"=6, "7"=7, "8"=8, "9"=9, "10"=10, "11"=11, "12"=12, "13"=13, "14"=14, "15"=15, "16"=16, "A (Control Input)"=17]
  in  "Channel2-2":u16(ring)=1 items=["1"=1, "2"=2, "3"=3, "4"=4, "5"=5, "6"=6, "7"=7, "8"=8, "9"=9, "10"=10, "11"=11, "12"=12, "13"=13, "14"=14, "15"=15, "16"=16, "A (Control Input)"=17]
  in  "Lakeshore 372 #6":bool
  in  "Calibration2-6":i32=6 min=0 max=32 step=1
  in  "Autorange2-6":bool
  in  "Lakeshore 372 #5":bool
  in  "Calibration2-5":i32=5 min=0 max=32 step=1
  in  "Autorange2-5":bool
  in  "Lakeshore 372 #4":bool
  in  "Calibration2-4":i32=4 min=0 max=32 step=1
  in  "Autorange2-4":bool
  in  "Lakeshore 372 #3":bool
  in  "Calibration2-3":i32=3 min=0 max=32 step=1
  in  "Autorange2-3":bool
  in  "Lakeshore 372 #2":bool
  in  "Calibration2-2":i32=2 min=0 max=32 step=1
  in  "Autorange2-2":bool
  in  "Lakeshore 372 #1":bool
  in  "Autoscan 2":bool
  in  "Calibration2-1":i32=1 min=0 max=32 step=1
  in  "Autorange2-1":bool
  in  "Change Pause Time (3) 2":dbl=3.0 min=3.0 max=200.0 step=1.0
  in  "Excitation On/Off (T: Excitation ON) 2":bool=TRUE
  in  "Configure (F:Don't Config) 2":bool
  in  "Channel On/Off (T: Channel ON) 2":bool=TRUE
  in  "Temperature Coefficient (0: Negative) 2":u16(ring) items=["Negative", "Positive"]
  in  "Excitation Mode (0: Voltage) 2":u16(ring) items=["Voltage", "Current"]
  in  "Scan Dwell Time (10) 2":dbl=10.0 min=1.0 max=200.0 step=1.0
  in  "VISA session LS372":refnum<visa-resource-name>="GPIB0::19::INSTR"
  in  "Set frequency through\ncommand file":bool=TRUE
  in  "AH 2700 Units":i32(ring)=1 items=["nanosiemens"=1, "dissipation factor"=2, "kilohms"=3, "gigohms"=4, "loss vector (jpF)"=5]
  in  "AH Maximum Voltage":dbl=15.0 min=0.0003 max=15.0 step=1.0 format="%#.6f"
  in  "AH Frequency":dbl(ring)=1000.0 items=["50"=50.0, "60"=60.0, "70"=70.0, "80"=80.0, "100"=100.0, "120"=120.0, "140"=140.0, "160"=160.0, "200"=200.0, "240"=240.0, "300"=300.0, "400"=400.0, "500"=500.0, "600"=600.0, "700"=700.0, "800"=800.0, "1000"=1000.0, "1200"=1200.0, "1400"=1400.0, "1600"=1600.0, "2000"=2000.0, "2400"=2400.0, "3000"=3000.0, "4000"=4000.0, "5000"=5000.0, "6000"=6000.0, "7000"=7000.0, "8000"=8000.0, "10000"=10000.0, "12000"=12000.0, "14000"=14000.0, "16000"=16000.0, "20000"=20000.0]
  in  "Average Exponent":u16=4 max=15
  in  "Visa AH 2700":refnum<visa-resource-name>
  out "Max y Field (T)":dbl=4.5
  out "Max z Field (T)":dbl=9.0
  out "Max Magnitude (T)":dbl=5.0
  in  "Box Adress":refnum<visa-resource-name>="COM4"
  out "Max Ramp Rate Z-Axis (A/s)":dbl=0.19
  out "Max Ramp Rate Y-Axis (A/s)":dbl=0.055
  in  "Z-Axis Communications Config":T9={"GPIB address"=22, "GPIB bus"=0, "connection ID"=refnum, "IP"="111.111.111.1", "Active Comm Interface"=0, "Serial Port"="", "Programmer Type"=0} {"Programmer Type" items=["Model 430", "Model 420"]; "Active Comm Interface" items=["TCP/IP (Model 430 Only)", "RS232", "IEEE488"]}
  in  "Y-Axis Communications Config":T9={"GPIB address"=22, "GPIB bus"=0, "connection ID"=refnum, "IP"="111.111.111.2", "Active Comm Interface"=0, "Serial Port"="", "Programmer Type"=0} {"Programmer Type" items=["Model 430", "Model 420"]; "Active Comm Interface" items=["TCP/IP (Model 430 Only)", "RS232", "IEEE488"]}
  in  "Configuration AMI135 (in)":T10={"Sensor Length (cm)"=66.0, "Hi Setpoint (cm)"=66.0, "Lo Setpoint (cm)"=33.0, "Sampling Interval (min)"=30.0} {"Sampling Interval (min)" min=0 max=600 format="%.1f"; "Lo Setpoint (cm)" min=0 max=203.2 format="%.1f"; "Hi Setpoint (cm)" min=0 max=203.2 format="%.1f"; "Sensor Length (cm)" min=1 max=203.2 format="%.1f"}
  in  "GPIB Setup Model 135":cluster{"GPIB address":i16, "GPIB bus":i16}={"GPIB address"=1, "GPIB bus"=0}
  in  "ILM Setup":T11={"Address"={"Com Port"=2, "ISOBUS Address"=6, "GPIB Address"=0, "Communication"=enum."ISOBUS"}, "ILM Name"="", "Display Channel"=[0]}
  in  "Lambda Controller Setup":T13={"Address"={"Com Port"=2, "ISOBUS Address"=3, "GPIB Address"=0, "Communication"=enum."ISOBUS"}, "Max 4.2K temp"=4.35, "Max 2.2K temp"=2.3} {"Max 2.2K temp" format="%.2f"; "Max 4.2K temp" format="%.2f"}
  in  "ITC Setup (new)":T14[](array[typedef])=[{"Description"="", "IO Info"={"Address"={"Com Port"=2, "ISOBUS Address"=1, "GPIB Address"=0, "Communication"=enum."ISOBUS"}, "Version"=enum."ITC503", "Ch 1 dec places"=0, "Ch 2 dec places"=0, "Ch 3 dec places"=0, "Ch1 Name"="", "Ch2 Name"="", "Ch3 Name"=""}}]
  in  "PSU Setup(read)":T17=[{"Max Sweep(4.2K)"=0.016666666666666666, "Max Sweep(2.2K)"=0.016666666666666666, "Switch htr dly"=30.0, "O/P contactor?"=FALSE, "Max Field(4.2K)"=14.0, "Max Field(2.2K)"=16.0, "Description\n"="IPS120-10  Version 3.07  (c) OXFORD 1996", "Settings.vi"=path "", "Max lead res"=0.5, "IO Info"={"Address"={"Com Port"=2, "ISOBUS Address"=2, "GPIB Address"=0, "Communication"=enum."ISOBUS"}, "Version"=enum."IPS"}, "Adjust shims"=FALSE}] {"Max lead res" format="%.2f"; "Max Field(2.2K)" format="%.2f"; "Max Field(4.2K)" format="%.2f"; "Switch htr dly" format="%.2f"; "Max Sweep(2.2K)" format="%.2f"; "Max Sweep(4.2K)" format="%.2f"}
  in  "Cluster":T20={"Mode"=enum."Immediate", "Bytes to Read"=5000, "IP Address"="172.25.187.107", "Remote Port"=33576, "Timeout"=10000}
  out "JT connection ID":refnum<k5>
  in  "Bin_file":refnum<file>
  in  "Bin_ini":refnum<file>
  in  "IO Info ITC":T15={"Address"={"Com Port"=2, "ISOBUS Address"=1, "GPIB Address"=24, "Communication"=enum."ISOBUS"}, "Version"=enum."ITC503", "Ch 1 dec places"=1, "Ch 2 dec places"=1, "Ch 3 dec places"=1, "Ch1 Name"="", "Ch2 Name"="", "Ch3 Name"=""}
  in  "ITC Info":T21={"ControlTITC"=0, "ControlTCh"=1, "SampleTITC"=0, "SampleTCh"=2}
  in  "IO Info IPS":T19={"Address"={"Com Port"=2, "ISOBUS Address"=2, "GPIB Address"=24, "Communication"=enum."ISOBUS"}, "Version"=enum."IPS"}
  in  "Stepsize (V)":dbl=1.0 min=0.0
  in  "Endwert (V)":dbl=6.0 min=-30.0 max=30.0 step=0.01
  in  "Startwert (V)":dbl=-6.0 min=-30.0 max=30.0 step=0.01
  in  "Messzeit [ms]":u32=7000
  in  "Delay [ms]":u32=10000
  # "Welcome to Sweet 16  High Precision Measurement Systems (S16HPMS)"
  # "LS370"
  # "Please Choose Insert:"
  # "Please Choose Instrument:"
  # "VTI"
  # "Measurement Info"
  # "Transport Sample  Parameters"
  # "Command-File Information and System Settings (usually not to change)"
  # "%"
  # "%"
  # "Lock In 1 setup"
  # "(s)"
  # "Lock In 2 setup"
  # "on\noff"
  # "on\noff"
  # "int\next"
  # "float\nground"
  # "AC\nDC"
  # "on\noff"
  # "on\noff"
  # "int\next"
  # "float\nground"
  # "AC\nDC"
  # "Keithley"
  # "Keithley 6221"
  # "Daten für Schnittstelle"
  # "Torque Probenstab Motor"
  # "In den Motor zu schreibende Daten"
  # "Lakeshore 370 - Thermometer Reading"
  # "Number of Datapoints\nstored in Monitor"
  # "Heater Setup"
  # "General"
  # "Ohm"
  # "Ohm"
  # "Ohm"
  # "Still / Channel 1"
  # "Temperature control"
  # "OFF"
  # "ON"
  # "OFF"
  # "ON"
  # "JT: Channel 4"
  # "(Default Sorb Channel: 2)"
  # "OFF"
  # "ON"
  # "OFF"
  # "ON"
  # "OFF"
  # "ON"
  # "OFF"
  # "ON"
  # "JT HX (3)"
  # "Achtung. IVC Plate ist CH 1\nauf LS370"
  # "OFF"
  # "ON"
  # "OFF"
  # "ON"
  # "IVC Plate (1)"
  # "ON"
  # "OFF"
  # "ON"
  # "OFF"
  # "Lakeshore 372 - Thermometer Reading"
  # "General"
  # "%"
  # "s"
  # "Channel 2"
  # "Channel 1"
  # "OFF"
  # "ON"
  # "OFF"
  # "ON"
  # "Channel 4"
  # "Channel 3"
  # "OFF"
  # "ON"
  # "OFF"
  # "ON"
  # "Channel 6"
  # "Channel 5"
  # "OFF"
  # "ON"
  # "OFF"
  # "ON"
  # "Capacity Bridge AH 2700"
  # "AMI Setup"
  # "IPS and ITC Adress Setup (Please no changes here)"
  # "Connection details JT"
  # "Hier werden Binärdateien mit datei-infos zum Init file, \nsowie zum  Mess-file gespeichert, \nda in der geupdateten Version von Windos, keine \nSpeicherung von Lokalen Variablen möglich ist.\n--> Fehler beim Öffnen der Binärdateien.\nDaher wird es jetzt im Instrument_Setup als Globale \nVariable gespeichert"
  # "Press Shift F1 to edit this field"
  # "ITC"
  # "Chan."
  # "Control temp."
  # "Sample temp."
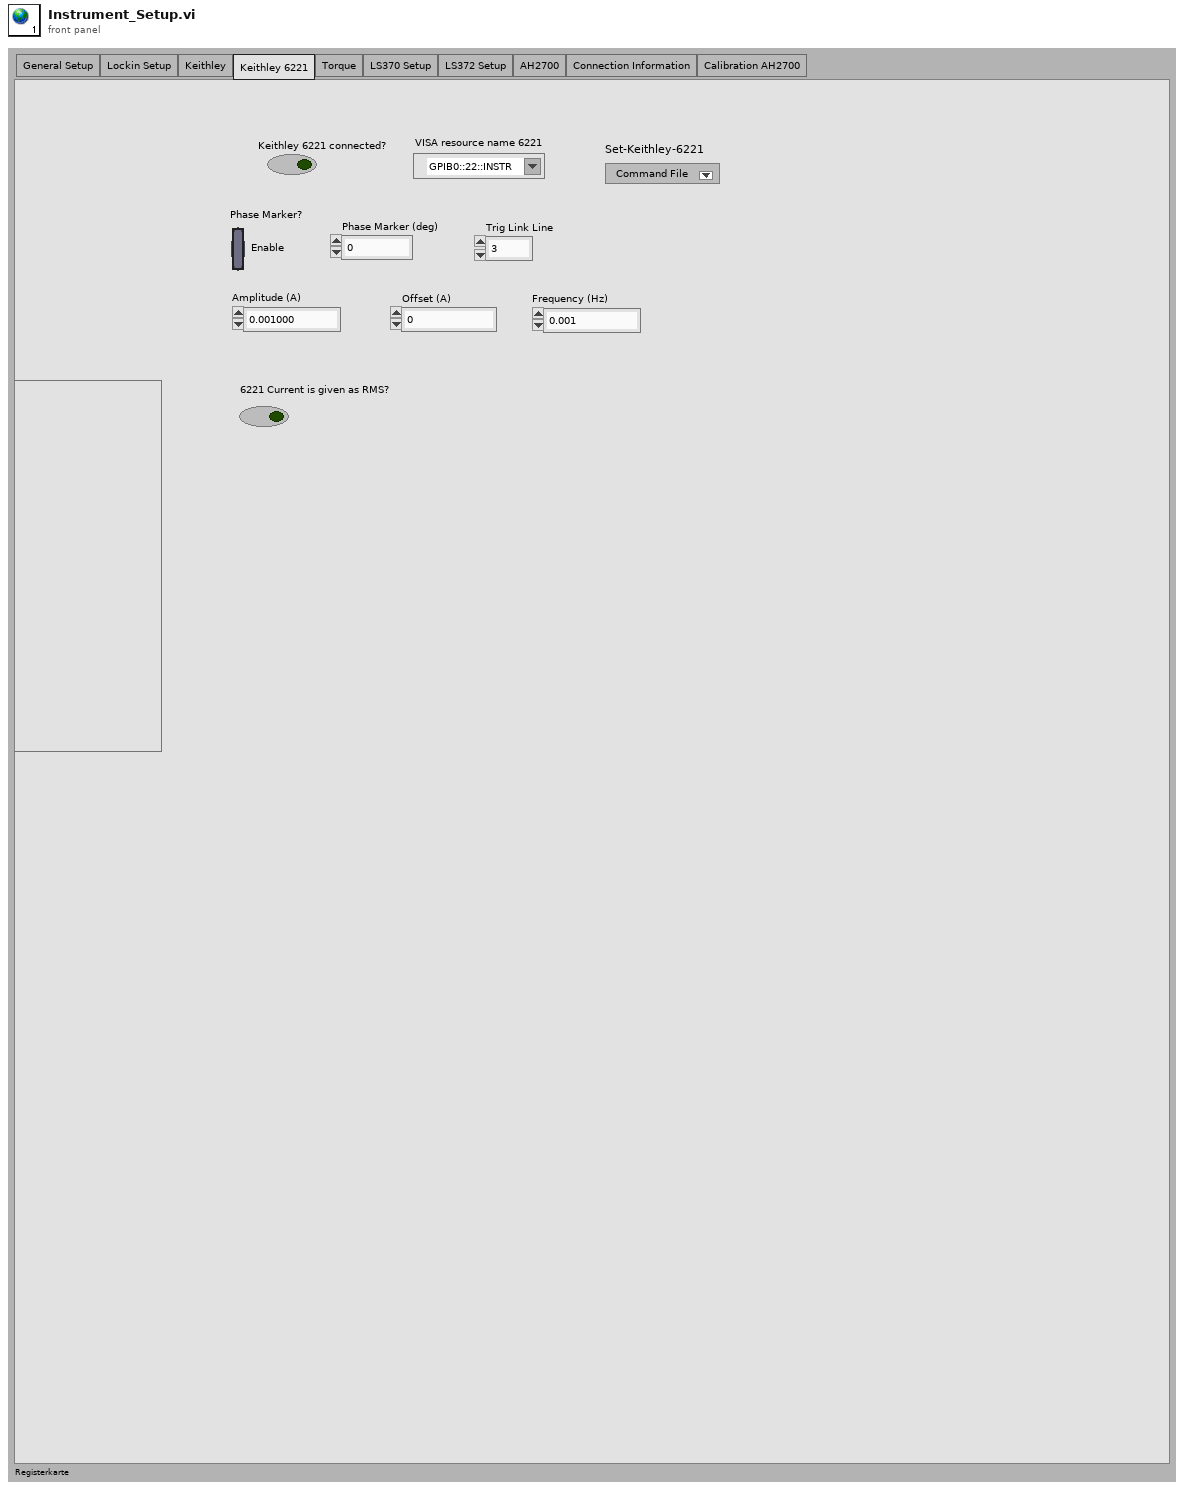
[diagram p1: front panel]
types:
  T1 = enum32{"Seite 1", "Lockin Setup", "Keithley", "Keithley 6221", "Torque", "LS370 Setup", "LS372 Setup", "AH2700", "Connection Information", "Calibration AH2700"}
  T2 = cluster{"time constant\n(10 µs : 0) ":i32, "slope (6 dB/oct)":i32}
  T3 = cluster{"sync filter":bool, "line filter\n(off:0)":i32}
  T4 = cluster{"sensitivity\n2nV/fA":i32, "dyn reserve\n(low noise:2)":i16, "ref. phase":ext, "automeasure":bool}
  T5 = cluster{"ref. source":bool, "osc.harm# ":u16, "osc. freq":ext, "osc. ampl.":ext, "ref. trigger":u16}
  T6 = cluster{"off. & exp.":u16, "offset":dbl, "expand":u16}
  T7 = cluster{"input":u16, "ground":bool, "couple":bool}
  T8 = cluster{" display":i32, " ratio":u16, "output":u16}
  T9 = cluster{"GPIB address":i16, "GPIB bus":i16, "connection ID":refnum<k5>, "IP":string, "Active Comm Interface":u16, "Serial Port":refnum<visa-resource-name>, "Programmer Type":u16}
  T10 = cluster{"Sensor Length (cm)":sgl, "Hi Setpoint (cm)":sgl, "Lo Setpoint (cm)":sgl, "Sampling Interval (min)":sgl}
  T11 = typedef "ILMSetup.ctl" = cluster{"Address":T12, "ILM Name":string, "Display Channel":i32[]}
  T12 = typedef "OxfordAddress.ctl" = cluster{"Com Port":i32, "ISOBUS Address":i32, "GPIB Address":i16, "Communication":enum16{"RS232", "ISOBUS", "GPIB", "Gateway"}}
  T13 = typedef "LambdaSetup.ctl" = cluster{"Address":T12, "Max 4.2K temp":dbl[unit], "Max 2.2K temp":dbl[unit]}
  T14 = typedef "ITCSetup.ctl" = cluster{"Description":string, "IO Info":T15}
  T15 = typedef "ITCIO.ctl" = cluster{"Address":T12, "Version":T16, "Ch 1 dec places":i16, "Ch 2 dec places":i16, "Ch 3 dec places":i16, "Ch1 Name":string, "Ch2 Name":string, "Ch3 Name":string}
  T16 = typedef "ITCVersion.ctl" = enum16{"ITC502", "ITC503", "ITC601"}
  T17 = typedef "PSSetupArray.ctl" = T18[]
  T18 = typedef "PSSetup.ctl" = cluster{"Max Sweep(4.2K)":dbl[unit], "Max Sweep(2.2K)":dbl[unit], "Switch htr dly":dbl[unit], "O/P contactor?":bool, "Max Field(4.2K)":dbl[unit], "Max Field(2.2K)":dbl[unit], "Description\n":string, "Settings.vi":path, "Max lead res":dbl[unit], "IO Info":T19, "Adjust shims":bool}
  T19 = typedef "PSIO.ctl" = cluster{"Address":T12, "Version":enum16{"PS", "IPS"}}
  T20 = cluster{"Mode":enum16{"Standard", "Buffered", "CRLF", "Immediate"}, "Bytes to Read":i32, "IP Address":string, "Remote Port":i32, "Timeout":i32}
  T21 = cluster{"ControlTITC":i8, "ControlTCh":i8, "SampleTITC":i8, "SampleTCh":i8}
diagram:
